vi "FileIO_Check_Directory_Exits_with_Write_Access.vi"(0 "Path In":path=path "\\\\itnas.appl.ge.com\\technology/Common/Software QA/Automation/Test Results", 5 "Free Space Required (Kb)":dbl=1000.0, 11 "Error Out":errorcluster) -> (4 "Path Out":path, 8 "Exists with Write Permissions ?":bool, 15 "Error In":errorcluster)   [LabVIEW 2016]
doc: "This VI will check thata particular folder exists, and that write acccess is granted."
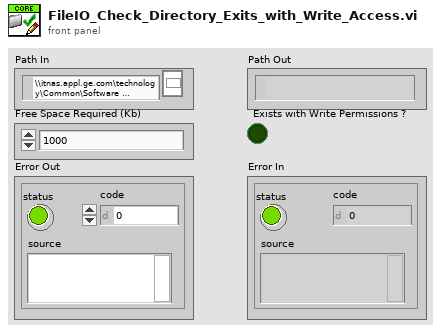
[diagram p1: front panel]
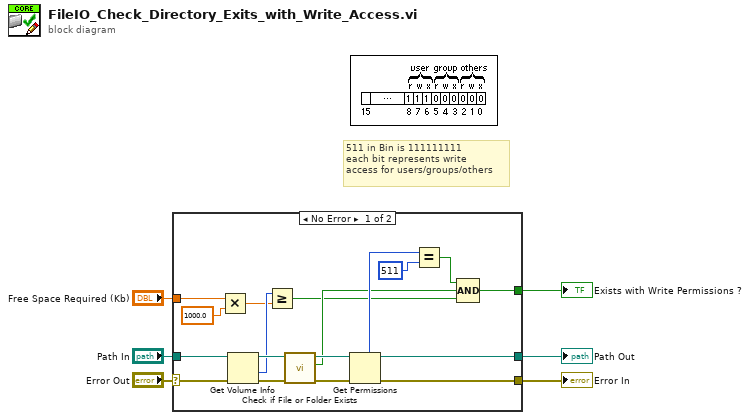
[diagram p0: block diagram]
diagram:
  # "511 in Bin is 111111111\neach bit represents write\naccess for users/groups/others"
  n1 = case shown="No Error" "Error Out" {
    selector: "Error Out" -> [w18 w26]
    tunnel: [w23 w26] -> w5
    tunnel: "Path In" -> [w16 w25]
    tunnel: [w21 w25] -> w3
    tunnel: [w12 _] -> w2
    tunnel: "Free Space Required (Kb)" -> [w8 _]
    frame No Error {
      n2 = Multiply(x=w8, y=1000.0) -> (x*y=w7:dbl)
      n3 = Get Volume Info(8:w18, 11:w16) -> (0:w17:errorcluster, 1:w14:i64, 3:w15:path)  [unwired: 3 out]
      n4 = Greater Or Equal?(x=w14, y=w7) -> (x >= y?=w10:bool)
      n5 = call <vilib>:"Check if File or Folder Exists.vi"("error in (no error)"=w17, "path"=w15) -> ("error out"=w24:errorcluster, "file or folder exists?"=w11:bool, "dup path"=w22:path)  [unwired: 7 in]
      n6 = Get Permissions(8:w24, 11:w22) -> (0:w23:errorcluster, 3:w21:path, 5:w20:i16)  [unwired: 2 out]
      n7 = Equal?(x=w20, y=i16 511) -> (x = y?=w13:bool)
      n8 = Compound Arithmetic op=AND(w13, w11, w10) -> (w12:bool)
    }
    frame Error {
    }
  }
  "Error In" <- w5
  "Exists with Write Permissions ?" <- w2
  "Path Out" <- w3
